vi "Tricon Send Command.vi"(7 "Address":u8, 8 "error in (no error)":errorcluster, 10 "Command":string, 11 "VISA resource name in":refnum<visa-resource-name>="COM3") -> (0 "error out":errorcluster, 1 "Status Code":string, 2 "Raw Response":string, 3 "VISA resource name out":refnum<visa-resource-name>, 4 "Value":dbl)   [LabVIEW 2018]
panel:
  out "error out 2":errorcluster
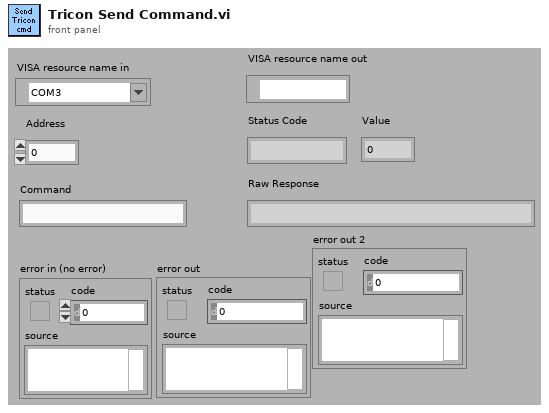
[diagram p1: front panel]
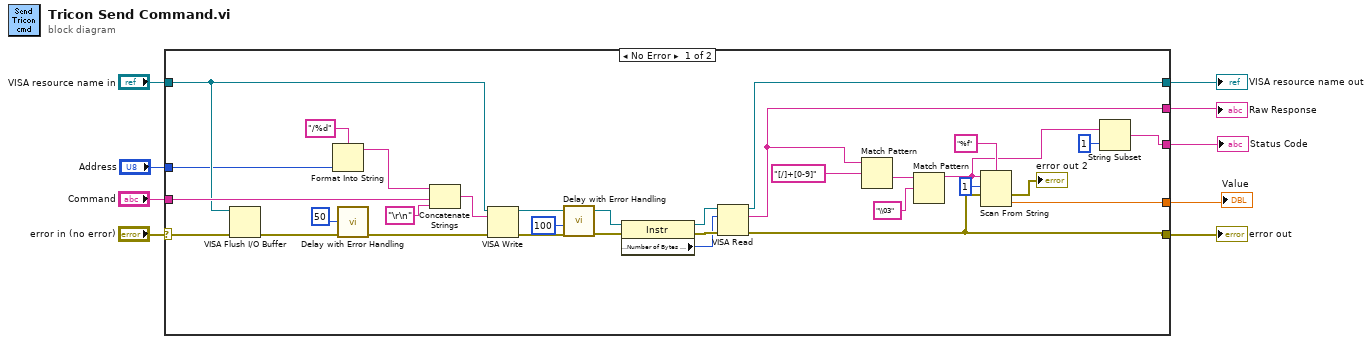
[diagram p0: block diagram]
diagram:
  n1 = case shown="No Error" "error in (no error)" {
    selector: "error in (no error)" -> [w25 w42]
    tunnel: "Command" -> [w29 _]
    tunnel: [w18 w42] -> w7
    tunnel: "VISA resource name in" -> [w23 w41]
    tunnel: [w34 w41] -> w5
    tunnel: [w19 _] -> w4
    tunnel: "Address" -> [w10 _]
    tunnel: [w15 _] -> w3
    tunnel: [w12 _] -> w2
    frame No Error {
      n2 = VISA Flush I/O Buffer(VISA resource name=w23, error in (no error)=w25) -> (error out=w24:errorcluster)  [unwired: 1 in, 1 out]
      n3 = Format Into String(format string="/%d", w10) -> (resulting string=w28:string)  [unwired: 2 in, 1 out]
      n4 = call "Delay with Error Handling.vi"("error in (no error)"=w24, "Delay (ms)"=u32 50) -> ("error out"=w26:errorcluster)  [unwired: 9 in]
      n5 = Concatenate Strings(w28, w29, "\r\n" ("string")) -> (w32:string)
      n6 = VISA Write(VISA resource name=w23, write buffer=w32, error in (no error)=w26) -> (VISA resource name out=w36:refnum<visa-resource-name>, error out=w40:errorcluster)  [unwired: 1 out]
      n7 = call "Delay with Error Handling.vi"("error in (no error)"=w40, "Delay (ms)"=u32 100) -> ("error out"=w38:errorcluster)  [unwired: 9 in]
      n8 = property class="Instr"(reference=w36, error in=w38) -> (reference out=w35:refnum<visa-resource-name>, error out=w37:errorcluster, "Serial Settings:Number of Bytes at Serial Port"=w33:u32)
      n9 = VISA Read(VISA resource name=w35, byte count=w33, error in (no error)=w37) -> (VISA resource name out=w34:refnum<visa-resource-name>, read buffer=w19:string, error out=w18:errorcluster)  [unwired: 1 out]
      n10 = Match Pattern(string=w19, regular expression="[/]+[0-9]") -> (after substring=w21:string)  [unwired: 1 in, 3 out]
      n11 = Match Pattern(string=w21, regular expression="\\03") -> (before substring=w11:string)  [unwired: 1 in, 3 out]
      n12 = Scan From String(format string="%f", input string=w11, initial scan location=u32 1, error in=w18) -> (error out=→"error out 2":errorcluster, output 1=w12:dbl)  [unwired: 1 in, 2 out]
      n13 = String Subset(string=w11, length (rest)=1 ("length (rest)")) -> (substring=w15:string)  [unwired: 1 in]
    }
    frame Error {
    }
  }
  "error out" <- w7
  "Raw Response" <- w4
  "VISA resource name out" <- w5
  "Status Code" <- w3
  "Value" <- w2
